vi "Uninitialize.vi"(8 "error in":errorcluster, 11 "TPCANHandle in":T1=81 items=["PCAN_NONEBUS"=0, "PCAN_USBBUS1"=81, "PCAN_USBBUS2"=82, "PCAN_USBBUS3"=83, "PCAN_USBBUS4"=84, "PCAN_USBBUS5"=85, "PCAN_USBBUS6"=86, "PCAN_USBBUS7"=87, "PCAN_USBBUS8"=88, "PCAN_USBBUS9"=1289, "PCAN_USBBUS10"=1290, "PCAN_USBBUS11"=1291, "PCAN_USBBUS12"=1292, "PCAN_USBBUS13"=1293, "PCAN_USBBUS14"=1294, "PCAN_USBBUS15"=1295, "PCAN_USBBUS16"=1296]) -> (0 "error out":errorcluster, 5 "TPCANStatus":u32)   [LabVIEW 2019, in "PCANBasic.lvlib"]
doc: "Uninitializes one or all PCAN Channels initialized by CAN_Initialize\nGiving the TPCANHandle value \"PCAN_NONEBUS\", \nuninitialize all initialized channels\n\nA PCAN Channel can be released using one of this possibilities: \n\nSingle-Release: Given a handle of a PCAN Channel initialized before with the method Initialize. If the given channel can not be found then an error is returned. \n\nMultiple-Release: Giving the handle value PCAN_NONEBUS which instructs the API to search for all channels initialized by the calling application and release them all. This option cause no errors if no hardware were uninitialized. \n\nTransmit-queue at uninitialize: When a PCAN-Basic channel connection is terminated, the underlying hardware's transmit-queue will not immediately be discarded. PCAN-Basic will wait some time before finalizing, so that the hardware has time to send (or try to send) those unsent messages. When the time is up (amount 500 milliseconds), the rest of the messages in the queue (if any) are discarded."
uses:
  PCANBasic.lvlib
  TPCANHandle.ctl
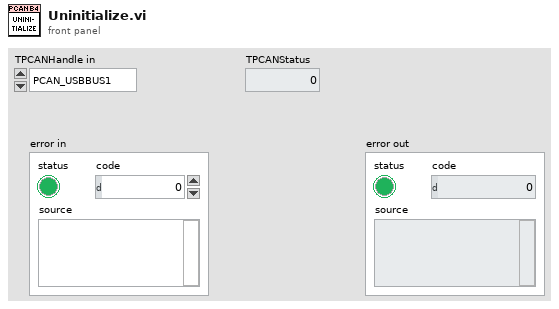
[diagram p1: front panel]
types:
  T1 = typedef "PCANBasic.lvlib/TPCANHandle.ctl" = u16
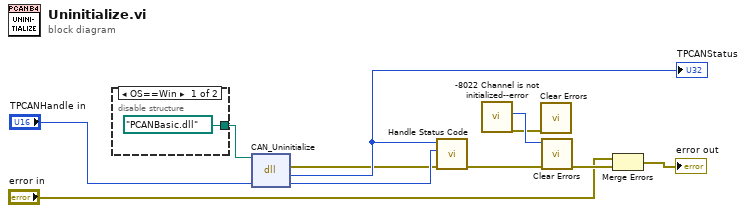
[diagram p0: block diagram]
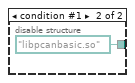
[diagram p2: hidden frame]
diagram:
  n1 = disable-structure shown="OS==Win" {
    disable-tunnel: [path "PCANBasic.dll" path "libpcanbasic.so"] -> w8
    frame condition #0 (active) {
    }
    frame condition #1 {
    }
  }
  n2 = dll-call lib="?" fn="CAN_Uninitialize"(path in=w8, "Channel"="TPCANHandle in") -> (error out=w2:errorcluster, "TPCANStatus"=w6:u32, "Channel"=w5:u16)  [unwired: 2 in, 1 out]
  "TPCANStatus" <- w6
  n3 = call "Handle Status Code.vi"("error in"=w2, "TPCANHandle"=w5, "TPCANStatus"=w6) -> ("error out"=w9:errorcluster)  [unwired: 8 in]
  n4 = call "-8022 Channel is not initialized--error.vi"() -> ("error out"=w1:errorcluster, "Error Code"=w11:i32)  [unwired: 10 in]
  n5 = call <vilib>:"Clear Errors.vi"("error in (no error)"=w1) -> ()  [unwired: 5 in, 2 out]
  n6 = call <vilib>:"Clear Errors.vi"("error in (no error)"=w9, "specific error code to clear (0: all)"=w11) -> ("error out"=w10:errorcluster)  [unwired: 4 in, 1 out]
  n7 = Merge Errors("error in", w10) -> (→"error out":errorcluster)
